vi "chooseDefensivePlay.vi"(8 "error in (no error)":errorcluster, 11 "Game in":refnum<class "Game.lvclass">) -> (0 "error out":errorcluster, 3 "Game out":refnum<class "Game.lvclass">)   [LabVIEW 2023, in "Game.lvclass"]
uses:
  Game.lvclass
  Game.lvclass/Game.ctl
  Team_class/Team.lvclass/Team.ctl
  Team_class/DefensivePlay.ctl
  NormalDefensiveWithDuelistPlay_class/NormalDefensiveWithDuelistPlay.lvclass
  Read DefensiveTeam.vi
  Team_class/Read DefensivePlay.vi
  Team_class/Write DefensivePlay.vi
  Write DefensiveTeam.vi
  Ally_class/Ally.lvclass
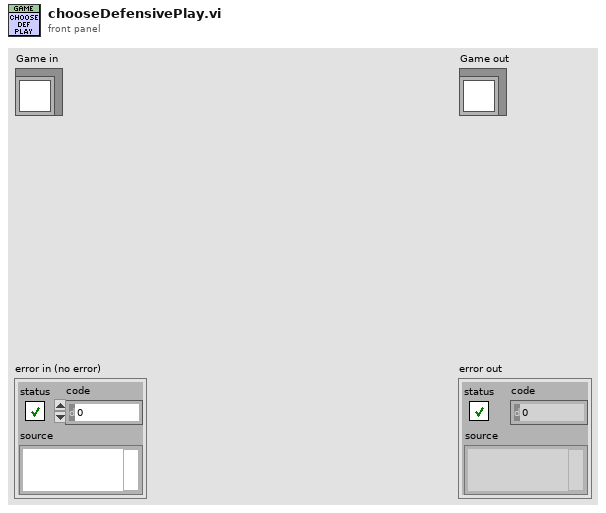
[diagram p1: front panel]
types:
  T1 = typedef "DefensivePlay.ctl" = enum16{"NormalDefensiveWithDuelist", "NormalDefensive", "TestPlay", "Halt", "Timeout", "PenaltyEnemy", "PenaltyAlly"}
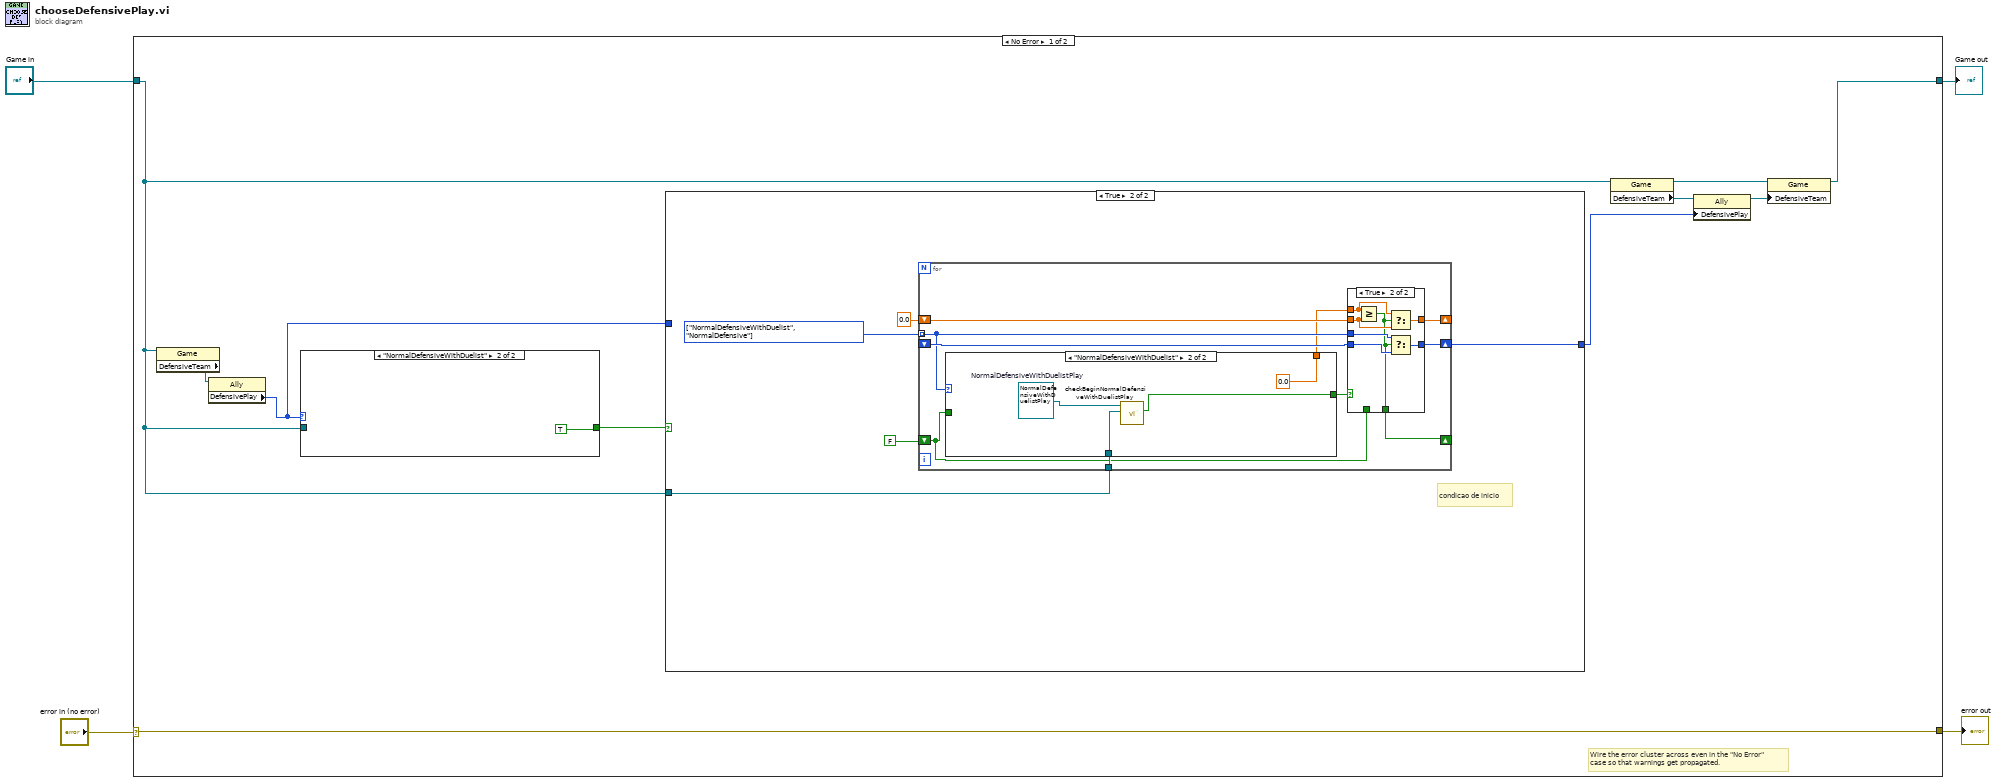
[diagram p0: block diagram]
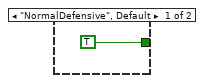
[diagram p2: hidden frame]
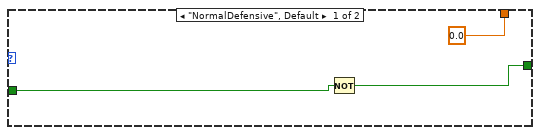
[diagram p4: hidden frame]
diagram:
  n1 = case shown="No Error" "error in (no error)" {
    selector: "error in (no error)" -> [w14 w51]
    tunnel: [w14 w51] -> w3
    tunnel: [w12 w50] -> w1
    tunnel: "Game in" -> [w5 w50]
    frame No Error {
      # "Wire the error cluster across even in the \"No Error\"\ncase so that warnings get propagated."
      n2 = property class="Game"(reference=w5) -> ("DefensiveTeam"=w11:refnum<class "Ally.lvclass">)  [unwired: 1 in, 2 out]
      n3 = property class="Ally"(reference=w11) -> ("DefensivePlay"=w9:T1)  [unwired: 1 in, 2 out]
      n4 = case shown="\"NormalDefensiveWithDuelist\"" w9 {
        tunnel: [TRUE TRUE] -> w10
        tunnel: w5 -> [_ _]
        frame "NormalDefensive", Default {
        }
        frame "NormalDefensiveWithDuelist" {
        }
      }
      n5 = case shown="True" w10 {
        tunnel: [w17 w21] -> w7
        tunnel: w9 -> [w17 _]
        tunnel: w5 -> [_ w19]
        frame False {
        }
        frame True {
          w20 = T1[] [enum."NormalDefensiveWithDuelist", enum."NormalDefensive"] items=["NormalDefensiveWithDuelist", "NormalDefensive", "TestPlay", "Halt", "Timeout", "PenaltyEnemy", "PenaltyAlly"] ("appended array")
          # "condicao de inicio"
          n6 = for {
            tunnel: w20 -> [w28] mode=indexing
            shift-right: [w31] -> _
            shift-left: 0.0 -> [w30]
            shift-right: [w29] -> w21
            shift-left: _ -> [w32]
            tunnel: w19 -> [w25]
            shift-right: [w24] -> _
            shift-left: FALSE -> [w23]
            n7 = case shown="\"NormalDefensiveWithDuelist\"" w28 {
              tunnel: [w34 w36] -> w27
              tunnel: [0.0 0.0] -> w26
              tunnel: w25 -> [_ w37]
              tunnel: w23 -> [w33 _]
              frame "NormalDefensive", Default {
                n8 = Not(x=w33) -> (.not. x?=w34:bool)
              }
              frame "NormalDefensiveWithDuelist" {
                w38 = refnum<class "NormalDefensiveWithDuelistPlay.lvclass"> refnum  # NormalDefensiveWithDuelistPlay
                n9 = call-dynamic "checkBeginNormalDefensiveWithDuelistPlay.vi"("Game"=w37, "NormalDefensiveWithDuelistPlay in"=w38) -> ("Duelist?"=w36:bool)  [unwired: 8 in, 1 out]
              }
            }
            n10 = case shown="True" w27 {
              tunnel: w32 -> [w41 w46]
              tunnel: [w42 w49] -> w31
              tunnel: w30 -> [w42 w45]
              tunnel: w28 -> [_ w47]
              tunnel: [w41 w48] -> w29
              tunnel: w26 -> [_ w44]
              tunnel: [w40 w43] -> w24
              tunnel: w23 -> [w40 _]
              frame False {
              }
              frame True {
                n11 = Greater Or Equal?(x=w44, y=w45) -> (x >= y?=w43:bool)
                n12 = Select(t=w44, s=w43, f=w45) -> (s? t:f=w49:dbl)
                n13 = Select(t=w47, s=w43, f=w46) -> (s? t:f=w48:T1)
              }
            }
          }
        }
      }
      n14 = property class="Game"(reference=w5) -> (reference out=w13:refnum<class "Game.lvclass">, "DefensiveTeam"=w8:refnum<class "Ally.lvclass">)  [unwired: 1 in, 1 out]
      n15 = property class="Ally"(reference=w8, "DefensivePlay"=w7) -> (reference out=w6:refnum<class "Ally.lvclass">)  [unwired: 1 in, 1 out]
      n16 = property class="Game"(reference=w13, "DefensiveTeam"=w6) -> (reference out=w12:refnum<class "Game.lvclass">)  [unwired: 1 in, 1 out]
    }
    frame Error {
    }
  }
  "error out" <- w3
  "Game out" <- w1
